vi "Structure Properties.vi"(0 "Length":i32, 2 "Width":i32, 3 "Height":i32) -> (5 "Inner Volume":i32, 6 "Volume":i32, 7 "Casing":i32, 8 "Inner Area":i32, 9 "Area":i32)   [LabVIEW 2024]
doc: "Calculate the volume and casing properties of a Mekanism multi-block structure."
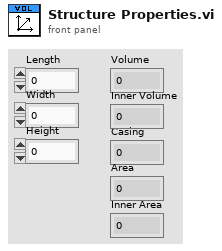
[diagram p1: front panel]
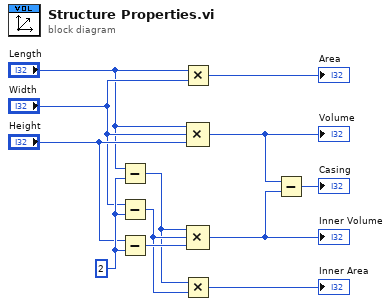
[diagram p0: block diagram]
diagram:
  w9 = 2
  n1 = Subtract(x="Length", y=w9) -> (x-y=w1:i32)
  n2 = Subtract(x="Width", y=w9) -> (x-y=w2:i32)
  n3 = Subtract(x="Height", y=w9) -> (x-y=w10:i32)
  n4 = Multiply(x="Length", y="Width") -> (x*y=→"Area":i32)
  n5 = Multiply(x=w1, y=w2) -> (x*y=→"Inner Area":i32)
  n6 = Compound Arithmetic op=MULTIPLY("Length", "Width", "Height") -> (w12:i32)
  "Volume" <- w12
  n7 = Compound Arithmetic op=MULTIPLY(w1, w2, w10) -> (w7:i32)
  "Inner Volume" <- w7
  n8 = Subtract(x=w12, y=w7) -> (x-y=→"Casing":i32)
